vi "get target by alias.vi"(8 "error in":errorcluster, 10 "alias":string, 11 "system hierarchy":T1) -> (0 "error out":errorcluster, 3 "target hierarchy":T1)   [LabVIEW 2013, in "PL_Serialization Interface.lvlib"]
uses:
  <vilib>/NI/Configuration Framework/tree serializer/flat hierarchy.ctl
  <vilib>/NI/Configuration Framework/tree serializer/full hierarchy.ctl
  <vilib>/NI/Configuration Framework/tree serializer/hierarchy element.ctl
  <vilib>/NI/Configuration Framework/tree serializer/instance data.ctl
  PL_Serialization Interface.lvlib
  <vilib>/NI/Configuration Framework/tree serializer/NISE_CEF_TreeSerializer.lvlib
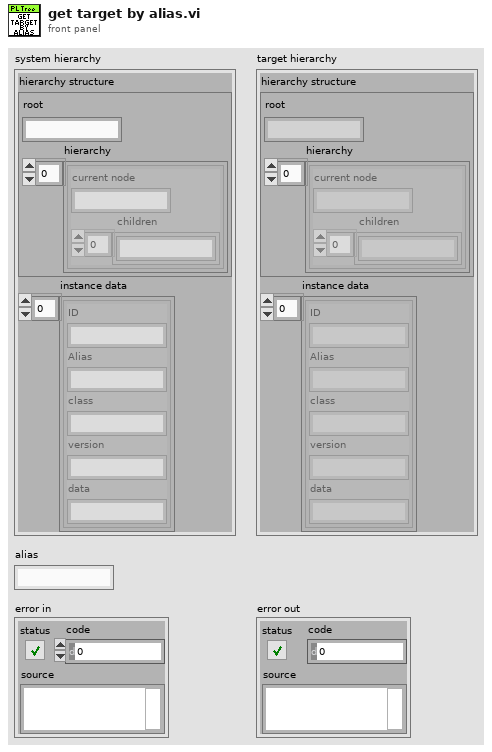
[diagram p1: front panel]
types:
  T1 = typedef "NISE_CEF_TreeSerializer.lvlib/flat hierarchy.ctl" = cluster{"hierarchy structure":T2, "instance data":T4[]}
  T2 = typedef "NISE_CEF_TreeSerializer.lvlib/full hierarchy.ctl" = cluster{"root":string, "hierarchy":T3[]}
  T3 = typedef "NISE_CEF_TreeSerializer.lvlib/hierarchy element.ctl" = cluster{"current node":string, "children":string[]}
  T4 = typedef "NISE_CEF_TreeSerializer.lvlib/instance data.ctl" = cluster{"ID":string, "Alias":string, "class":string, "version":string, "data":string}
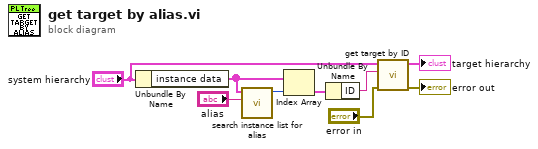
[diagram p0: block diagram]
diagram:
  n1 = Unbundle By Name("system hierarchy") -> ("instance data"=w6:T4[])
  n2 = call <vilib>:"search instance list for alias.vi"("alias"="alias", "instance data"=w6) -> ("index"=w9:i32)  [unwired: 9 in]
  n3 = Index Array(array=w6, index=w9) -> (element=w5:T4)
  n4 = Unbundle By Name(w5) -> ("ID"=w4:string)
  n5 = call "get target by ID.vi"("error in"="error in", "UID"=w4, "full system"="system hierarchy") -> ("error out"=→"error out":errorcluster, "target hierarchy"=→"target hierarchy":T1)  [unwired: 7 in]
